vi "Variant to Reply String.vi"(8 "error in (no error)":errorcluster, 9 "Data":variant, 11 "Instrument.1820 in":refnum<class "Instrument.Oxford1820.lvclass">) -> (0 "error out":errorcluster, 1 "Reply":string, 3 "Instrument.1820 out":refnum<class "Instrument.Oxford1820.lvclass">)   [LabVIEW 2016, in "Instrument.Oxford1820.lvclass"]
uses:
  Instrument.Oxford1820.lvclass
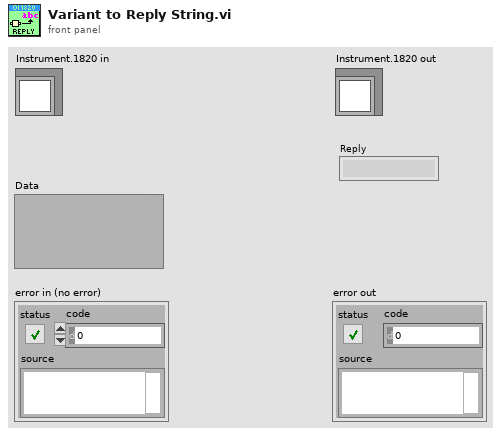
[diagram p1: front panel]
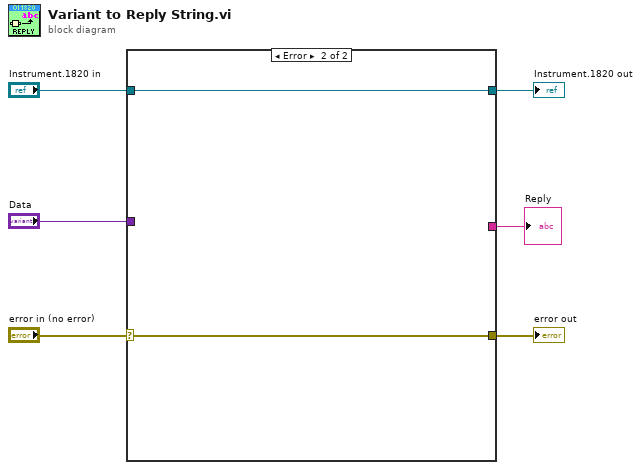
[diagram p0: block diagram]
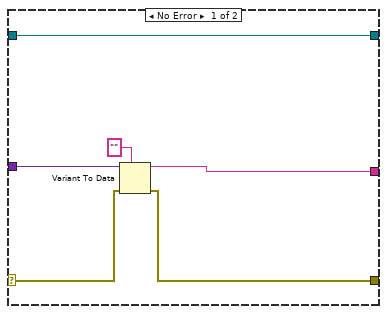
[diagram p2: hidden frame]
diagram:
  n1 = case shown="Error" "error in (no error)" {
    selector: "error in (no error)" -> [w10 w14]
    tunnel: "Data" -> [w9 _]
    tunnel: [w8 w14] -> w5
    tunnel: "Instrument.1820 in" -> [w12 w13]
    tunnel: [w12 w13] -> w2
    tunnel: [w7 _] -> w1
    frame No Error {
      n2 = Variant To Data(error in=w10, type="", Variant=w9) -> (data=w7:string, error out=w8:errorcluster)
    }
    frame Error {
    }
  }
  "Instrument.1820 out" <- w2
  "error out" <- w5
  "Reply" <- w1
